vi "STS_Add_Ref_MonitorData.vi"(7 "setting":refnum<k24>, 8 "错误输入（无错误）":errorcluster, 9 "monitorData":sgl[](array[numeric]), 10 "triggerIndex":sgl[](array[numeric]), 11 "STSProcess.ILSTS":refnum<k24>) -> (0 "错误输出":errorcluster, 3 "ILSTS out":refnum<k24>)   [LabVIEW 2017]
uses:
  D:/test/ILSTS/LV_IL_Sample/DLL/STSProcess.dll
  DLL/STSProcess.dll
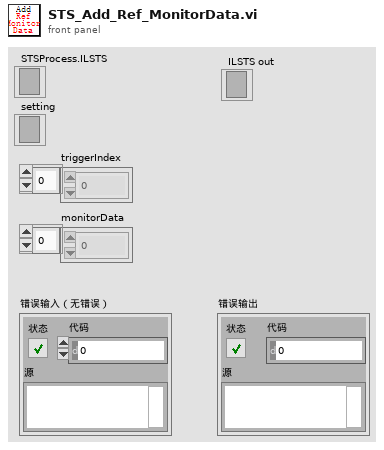
[diagram p1: front panel]
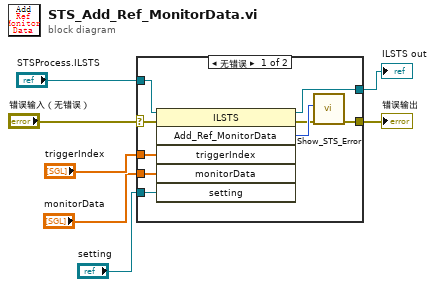
[diagram p0: block diagram]
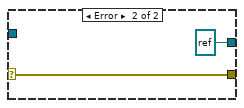
[diagram p2: hidden frame]
diagram:
  n1 = case shown="无错误" "错误输入（无错误）" {
    selector: "错误输入（无错误）" -> [w15 w18]
    tunnel: [w11 w18] -> w7
    tunnel: "STSProcess.ILSTS" -> [w16 _]
    tunnel: [w14 refnum<k24> refnum ("STSProcess.ILSTS")] -> w4
    tunnel: "setting" -> [w10 _]
    tunnel: "triggerIndex" -> [w9 _]
    tunnel: "monitorData" -> [w8 _]
    frame No Error {
      n2 = invoke on="调用节点" class="ILSTS" method="Add_Ref_MonitorData"(reference=w16, error in=w15, "triggerIndex"=w9, "monitorData"=w8, "setting"=w10) -> (reference out=w14:refnum<k24>, error out=w12:errorcluster, "Add_Ref_MonitorData"=w13:i32)  [unwired: 1 in, 3 out]
      n3 = call "Show_STS_Error.vi"("error in (no error)"=w12, "Error"=w13) -> ("error out"=w11:errorcluster)  [unwired: 9 in]
    }
    frame Error {
    }
  }
  "错误输出" <- w7
  "ILSTS out" <- w4
